vi "S2C_VAR_MenuLoad.vi"(8 "Error In":errorcluster, 9 "Coords":T1, 10 "MenuRef":refnum<k9>, 11 "CtrlRef":refnum<vi>) -> (0 "Error Out":errorcluster, 3 "Discard?":bool)   [LabVIEW 2015]
uses:
  <vilib>/Utility/miscctls.llb/LVPoint32TypeDef.ctl
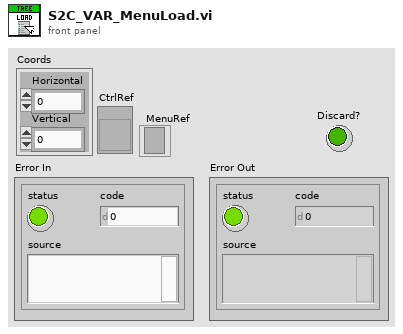
[diagram p1: front panel]
types:
  T1 = typedef "LVPoint32TypeDef.ctl" = cluster{"Horizontal":i32, "Vertical":i32}
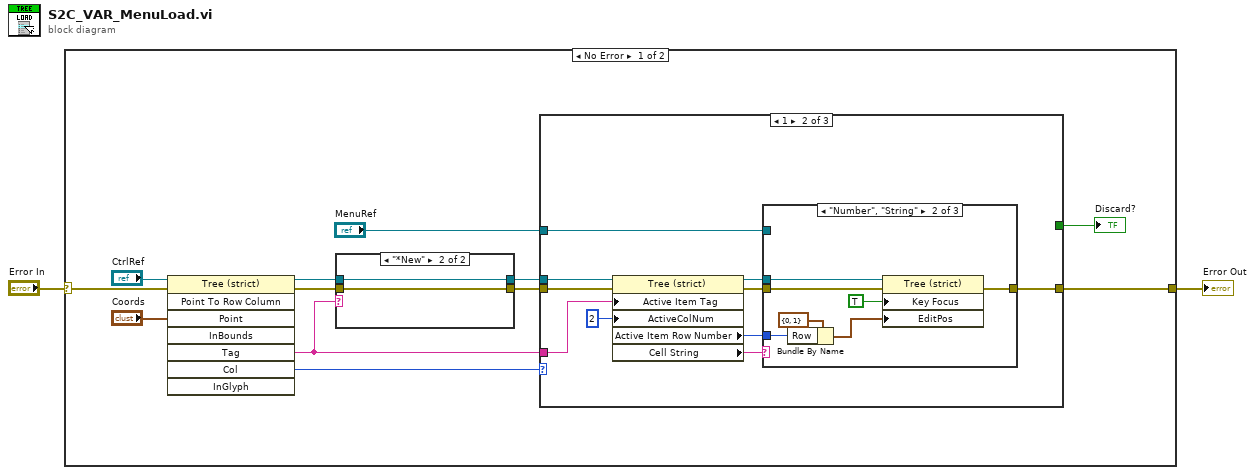
[diagram p0: block diagram]
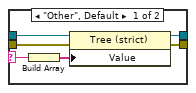
[diagram p2: hidden frame]
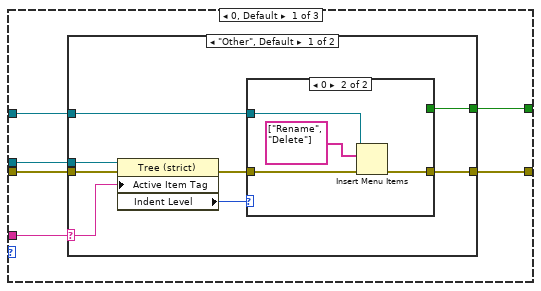
[diagram p3: hidden frame]
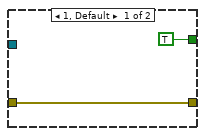
[diagram p4: hidden frame]
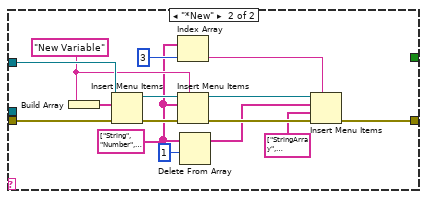
[diagram p5: hidden frame]
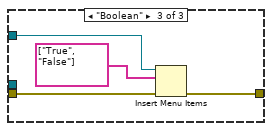
[diagram p7: hidden frame]
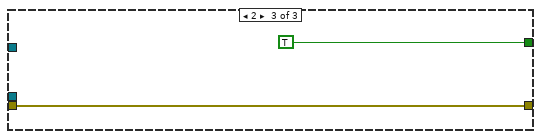
[diagram p8: hidden frame]
diagram:
  n1 = case shown="No Error" "Error In" {
    selector: "Error In" -> [w12 w82]
    tunnel: [w4 w82] -> w1
    frame No Error {
      n2 = invoke on="Invoke Node" class="Tree (strict)" method="Point To Row Column"(reference="CtrlRef", error in=w12, "Point"="Coords") -> (reference out=w9:refnum<vi>, error out=w14:errorcluster, "Tag"=w8:string, "Col"=w7:i32)  [unwired: 5 in, 4 out]
      n3 = case shown="\"*New\"" w8 {
        selector: w8 -> [w17 _]
        tunnel: w14 -> [w20 w22]
        tunnel: [w18 w22] -> w13
        tunnel: w9 -> [w16 w21]
        tunnel: [w15 w21] -> w6
        frame "Other", Default {
          n4 = Build Array(w17) -> (w19:string[])
          n5 = property on="Property Node" class="Tree (strict)"(reference=w16, error in=w20, "Value"=w19) -> (reference out=w15:refnum<vi>, error out=w18:errorcluster)
        }
        frame "*New" {
        }
      }
      n6 = case shown="1" w7 {
        tunnel: w8 -> [w28 w66 _]
        tunnel: w13 -> [w27 w67 w81]
        tunnel: [w26 _ TRUE] -> w3
        tunnel: [w25 w63 w81] -> w4
        tunnel: "MenuRef" -> [w24 w60 _]
        tunnel: w6 -> [w23 w59 _]
        frame 0, Default {
          n7 = case shown="\"Other\", Default" w28 {
            selector: w28 -> [w33 _]
            tunnel: w27 -> [w34 w57]
            tunnel: [w30 _] -> w26
            tunnel: [w35 w44] -> w25
            tunnel: w24 -> [w36 w56]
            tunnel: w23 -> [w29 _]
            frame "Other", Default {
              n8 = property on="Property Node" class="Tree (strict)"(reference=w29, error in=w34, "Active Item Tag"=w33) -> (error out=w32:errorcluster, "Indent Level"=w31:i32)  [unwired: 1 out]
              n9 = case shown="0" w31 {
                tunnel: w36 -> [_ w42]
                tunnel: [w38 w41] -> w35
                tunnel: w32 -> [w38 w40]
                tunnel: [TRUE _] -> w30
                frame 1, Default {
                }
                frame 0 {
                  n10 = Insert Menu Items(6:w40, 8:string[] ["Rename", "Delete"], 9:w42) -> (0:w41:errorcluster)  [unwired: 3 in, 2 out]
                }
              }
            }
            frame "*New" {
              w47 = string[] ["String", "Number", "Boolean", "Array"]
              w53 = "New Variable"
              n11 = Build Array(w53) -> (w55:string[])
              n12 = Insert Menu Items(6:w57, 8:w55, 9:w56) -> (0:w54:errorcluster, 3:w51:refnum<k9>)  [unwired: 3 in, 1 out]
              n13 = Index Array(array=w47, index=3) -> (element=w48:string)
              n14 = Insert Menu Items(5:w53, 6:w54, 8:w47, 9:w51) -> (0:w52:errorcluster, 3:w50:refnum<k9>)  [unwired: 2 in, 1 out]
              n15 = Delete From Array(array=w47, length=1) -> (array with subset deleted=w45:string[])  [unwired: 1 in, 1 out]
              n16 = Insert Menu Items(5:w48, 6:w52, 7:string[] ["StringArray", "NumberArray", "BooleanArray"], 8:w45, 9:w50) -> (0:w44:errorcluster)  [unwired: 1 in, 2 out]
            }
          }
        }
        frame 1 {
          n17 = property on="Property Node" class="Tree (strict)"(reference=w59, error in=w67, "Active Item Tag"=w66, "ActiveColNum"=2 ("Active Cell:Active Column Number")) -> (reference out=w58:refnum<vi>, error out=w64:errorcluster, "Active Item Row Number"=w61:i32, "Cell String"=w62:string)
          n18 = case shown="\"Number\", \"String\"" w62 {
            tunnel: w64 -> [w68 w75 w79]
            tunnel: [w68 w74 w76] -> w63
            tunnel: w61 -> [_ w72 _]
            tunnel: w60 -> [_ _ w78]
            tunnel: w58 -> [_ w69 _]
            frame "Other", Default {
            }
            frame "Number", "String" {
              n19 = Bundle By Name(cluster=cluster{"Row":i32, "Column":i32} {"Row"=0, "Column"=1} ("Edit Position"), "Row"=w72) -> (w71:cluster{"Row":i32, "Column":i32})
              n20 = property on="Property Node" class="Tree (strict)"(reference=w69, error in=w75, "Key Focus"=TRUE, "EditPos"=w71) -> (error out=w74:errorcluster)  [unwired: 1 out]
            }
            frame "Boolean" {
              n21 = Insert Menu Items(6:w79, 8:string[] ["True", "False"], 9:w78) -> (0:w76:errorcluster)  [unwired: 3 in, 2 out]
            }
          }
        }
        frame 2 {
        }
      }
      "Discard?" <- w3
    }
    frame Error {
    }
  }
  "Error Out" <- w1
